vi "XLP80_Action_StartTestmode_B.vi"(8 "err in":errorcluster) -> (0 "err out":errorcluster)   [LabVIEW 2021]
uses:
  XLP80_FGlob/1886_FGlob_TDefs_Enum_FGlobItems.ctl
  XLP80_FGlob/1886_FGlob_TDefEnumCANWriteItems.ctl
  XLP80_State_V001.llb/XLP80_State_Globals.vi
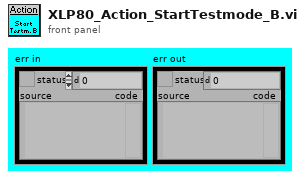
[diagram p1: front panel]
types:
  T1 = typedef "1886_FGlob_TDefs_Enum_FGlobItems.ctl" = enum16{"Put one", "Put all", "Recall one", "Recall all"}
  T2 = typedef "1886_FGlob_TDefEnumCANWriteItems.ctl" = enum16{"LV_Testmode_Select", "LV_A_71_Current_Out_Set", "LV_A_71_Voltage_In_Set", "LV_A_71_Voltage_Out_Set", "LV_H_51_STK_CellVoltages_Enable", "S80_BP_s_Taster_Start_Status"}
  T3 = typedef "XLP80_State_TDefEnumGlobalState.ctl" = enum16{"HV & Software", "Basis Funktion", "Power Management", "Operational Mode", "Shutdown", "Alarm"}
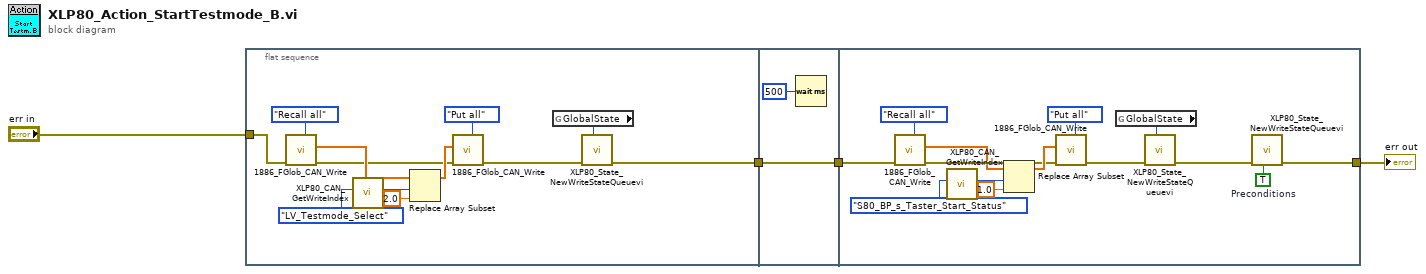
[diagram p0: block diagram]
diagram:
  n1 = flat-sequence {
    tunnel: "err in" -> [w9]
    tunnel: [w6] -> w1
    tunnel: [w17] -> w3
    tunnel: w1 -> [w17]
    tunnel: [w20] -> w4
    tunnel: w3 -> [w26]
    frame #0 {
      n2 = call "1886_FGlob_CAN_Write.vi"("Function (Recall One)"=1886_FGlob_TDefs_Enum_FGlobItems."Recall all", "err in"=w9) -> ("err out"=w8:errorcluster, "AO Values OUT"=w11:dbl[])  [unwired: 7 in, 1 out]
      n3 = call "XLP80_CAN_GetWriteIndex.vi"("CAN Write Items"=1886_FGlob_TDefEnumCANWriteItems."LV_Testmode_Select" ("CAN Write Items Testmode_A")) -> ("Index"=w14:i32)  [unwired: 10 in]
      n4 = Replace Array Subset(array=w11, new element=2.0 ("new element/subarray"), index=w14) -> (w10:dbl[])
      n5 = call "1886_FGlob_CAN_Write.vi"("Function (Recall One)"=1886_FGlob_TDefs_Enum_FGlobItems."Put all", "err in"=w8, "AO Values IN"=w10) -> ("err out"=w7:errorcluster)  [unwired: 6 in, 2 out]
      n6 = global read "XLP80_State_Globals.vi" "GlobalState"() -> (w5:T3)
      n7 = call "XLP80_State_NewWriteStateQueuevi.vi"("GlobalState"=w5, "err in"=w7) -> ("err out"=w6:errorcluster)  [unwired: 9 in]
    }
    frame #1 {
      n8 = Wait (ms)(milliseconds to wait=u32 500) -> ()  [unwired: 1 out]
    }
    frame #2 {
      w19 = TRUE  # Preconditions
      n9 = call "1886_FGlob_CAN_Write.vi"("Function (Recall One)"=1886_FGlob_TDefs_Enum_FGlobItems."Recall all", "err in"=w26) -> ("err out"=w25:errorcluster, "AO Values OUT"=w24:dbl[])  [unwired: 7 in, 1 out]
      n10 = call "XLP80_CAN_GetWriteIndex.vi"("CAN Write Items"=1886_FGlob_TDefEnumCANWriteItems."S80_BP_s_Taster_Start_Status" ("CAN Write Items Testmode_A")) -> ("Index"=w29:i32)  [unwired: 10 in]
      n11 = Replace Array Subset(array=w24, new element=1.0 ("new element/subarray"), index=w29) -> (w32:dbl[])
      n12 = call "1886_FGlob_CAN_Write.vi"("Function (Recall One)"=1886_FGlob_TDefs_Enum_FGlobItems."Put all", "err in"=w25, "AO Values IN"=w32) -> ("err out"=w22:errorcluster)  [unwired: 6 in, 2 out]
      n13 = global read "XLP80_State_Globals.vi" "GlobalState"() -> (w23:T3)
      n14 = call "XLP80_State_NewWriteStateQueuevi.vi"("GlobalState"=w23, "err in"=w22) -> ("err out"=w21:errorcluster)  [unwired: 9 in]
      n15 = call "XLP80_State_NewWriteStateQueuevi.vi"("Preconditions"=w19, "err in"=w21) -> ("err out"=w20:errorcluster)  [unwired: 9 in]
    }
  }
  "err out" <- w4
